vi "Day 4-1.vi"() -> ()   [LabVIEW 2019, in "Day 4.lvlib"]
uses:
  Day 4.lvlib
panel:
  out "Result":i32
  out "Winner Turn Number":i32
  out "Winner Board Status":bool[][](array[boolean])
  out "Winner Board":i32[][](array[numeric])
  out "Matrices":i32[][][](array[numeric])
  out "Turns Numbers":i32[](array[numeric])
  in  "String":string="124\n125\n127\n128\n132\n140\n142\n103\n102\n110\n101\n107\n109\n113\n119\n120\n122\n124\n125\n121\n119\n139\n159\n164\n165\n177\n190\n181\n182\n171\n192\n185\n184\n186\n183\n203\n204\n209\n210\n214\n215\n213\n235\n257\n271\n278\n279\n284\n286\n289\n290\n287\n291\n297\n287\n290\n273\n280\n284\n288\n289\n294\n310\n324\n319\n320\n324\n325\n327\n328\n326\n328\n300\n301\n302\n306\n308\n315\n349\n364\n365\n367\n369\n376\n384\n386\n378\n382\n396\n427\n435\n434\n437\n424\n432\n443\n453\n451\n453\n440\n446\n447\n448\n449\n454\n462\n463\n448\n447\n448\n460\n468\n469\n470\n473\n479\n480\n481\n488\n498\n499\n502\n504\n510\n513\n507\n506\n504\n507\n518\n520\n519\n515\n520\n536\n534\n535\n537\n554\n555\n556\n558\n554\n566\n558\n542\n545\n552\n556\n563\n..."
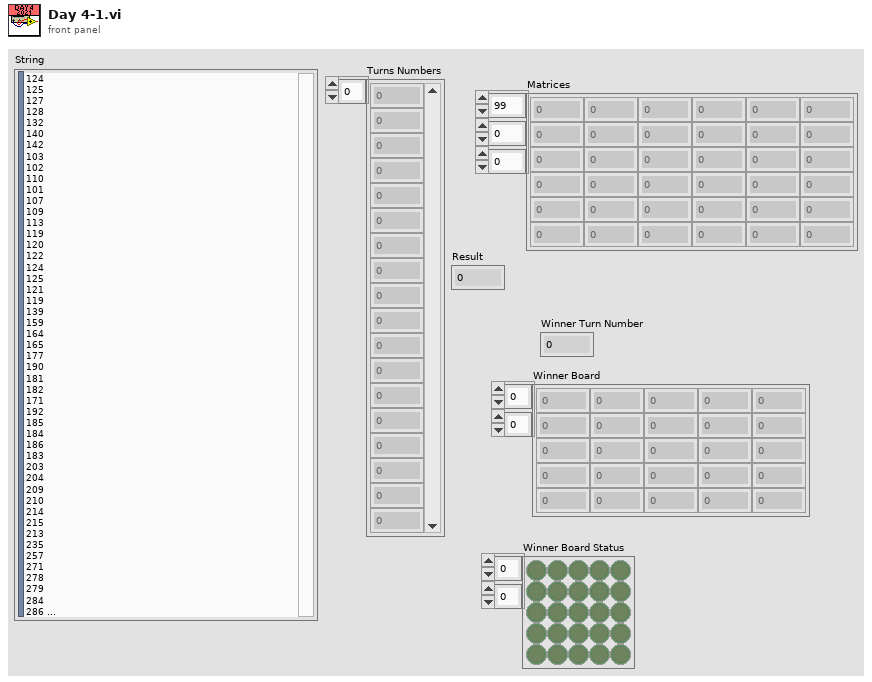
[diagram p1: front panel]
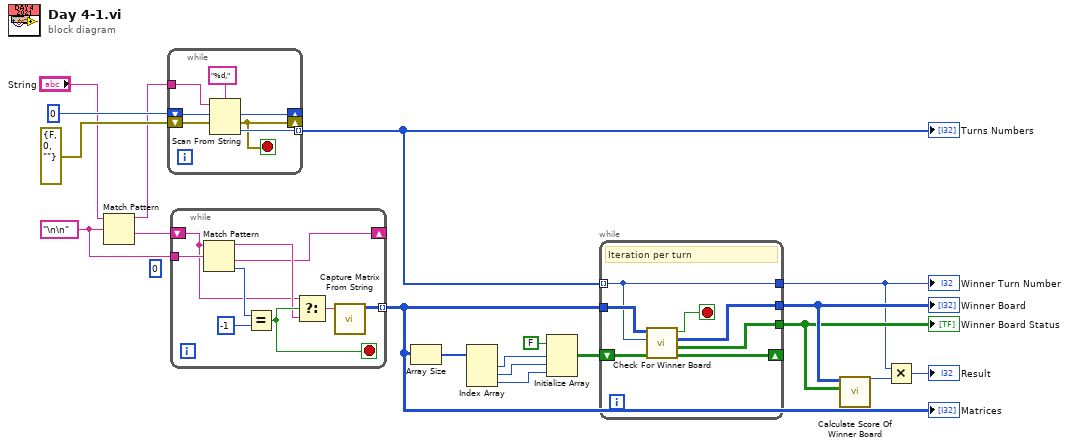
[diagram p0: block diagram]
diagram:
  (unwired) 0 ("offset past match")
  w14 = "\n\n" ("regular expression")
  n1 = Match Pattern(string="String", regular expression=w14) -> (before substring=w16:string, after substring=w15:string)  [unwired: 1 in, 2 out]
  n2 = while {
    tunnel: [w24] -> w13 mode=indexing
    tunnel: w16 -> [w26]
    shift-right: [w21] -> _
    shift-left: u32 0 -> [w23]
    shift-right: [w20] -> _
    shift-left: errorcluster {"status"=FALSE, "code"=0, "source"=""} ("error IO") -> [w22]
    stop <- w20 stop-if-true
    n3 = Scan From String(format string="%d,", input string=w26, initial scan location=w23, error in=w22) -> (offset past scan=w21:u32, error out=w20:errorcluster, output 1=w24:i32)  [unwired: 1 in, 1 out]
  }
  "Turns Numbers" <- w13
  n4 = while {
    tunnel: w14 -> [w35]
    tunnel: [w32] -> w11 mode=indexing
    shift-right: [w29] -> _
    shift-left: w15 -> [w27]
    stop <- w33 stop-if-true
    n5 = Match Pattern(string=w27, regular expression=w35) -> (before substring=w30:string, after substring=w29:string, offset past match=w31:i32)  [unwired: 1 in, 1 out]
    n6 = Equal?(x=w31, y=-1) -> (x = y?=w33:bool)
    n7 = Select(t=w27, s=w33, f=w30) -> (s? t:f=w28:string)
    n8 = call "Capture Matrix From String.vi"("String"=w28) -> ("Array"=w32:i32[][])  [unwired: 10 in]
  }
  "Matrices" <- w11
  n9 = Array Size(array=w11) -> (size(s)=w10:i32[])
  n10 = Index Array(array=w10) -> (element #1=w9:i32, element #2=w8:i32, element #3=w7:i32)  [unwired: 3 in]
  n11 = Initialize Array(FALSE, w9, w8, w7) -> (w6:bool[][][])
  n12 = while {
    tunnel: w13 -> [w36] mode=indexing
    tunnel: w11 -> [w42]
    shift-right: [w40] -> _
    shift-left: w6 -> [w41]
    tunnel: [w38] -> w5
    tunnel: [w37] -> w4
    tunnel: [w36] -> w2
    stop <- w39 stop-if-true
    # "Iteration per turn"
    n13 = call "Check For Winner Board.vi"("Matrixes Status In"=w41, "Turn Number"=w36, "Boards"=w42) -> ("Matrixes Status Out"=w40:bool[][][], "Winner Board Status"=w37:bool[][], "Winner Board"=w38:i32[][], "Winner Found?"=w39:bool)  [unwired: 5 in]
  }
  "Winner Board" <- w5
  "Winner Board Status" <- w4
  "Winner Turn Number" <- w2
  n14 = call "Calculate Score Of Winner Board.vi"("Winner Board Status"=w4, "Winner Board"=w5) -> ("Score"=w3:i32)  [unwired: 9 in]
  n15 = Multiply(x=w2, y=w3) -> (x*y=→"Result":i32)
